vi "DestroyClone.vi"(8 "error in (no error)":errorcluster, 9 "Exit via Stop Module Req?":bool, 10 "Wait for Module to stop?":bool, 11 "ModuleAdmin":refnum<class "ModuleAdmin.lvclass">) -> (0 "error out":errorcluster, 1 "External Launch":bool, 3 "Mod Admin out":refnum<class "ModuleAdmin.lvclass">)   [LabVIEW 2014, in "FGenModule.lvlib"]
uses:
  FGenModule.lvlib
  <userlib>/NIST/ModuleAdminLib/ModuleAdmin/ModuleAdmin.lvclass
  <userlib>/NIST/ModuleAdminLib/ModuleAdmin/ModuleAdmin.lvclass/ModuleAdmin.ctl
  <userlib>/NIST/ModuleAdminLib/ModuleAdmin/Accessors/Read CloneRegRef.vi
  <userlib>/NIST/ModuleAdminLib/CloneRegistration/CloneRegistration.lvclass
  <userlib>/NIST/ModuleAdminLib/ModuleAdminBase/ModuleAdminBase.lvclass
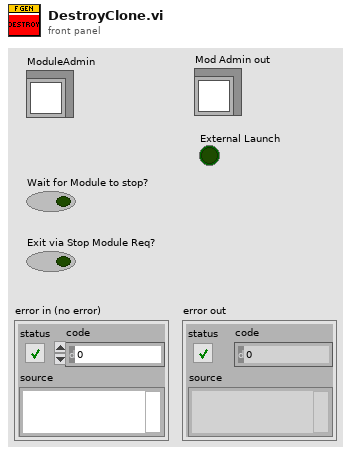
[diagram p1: front panel]
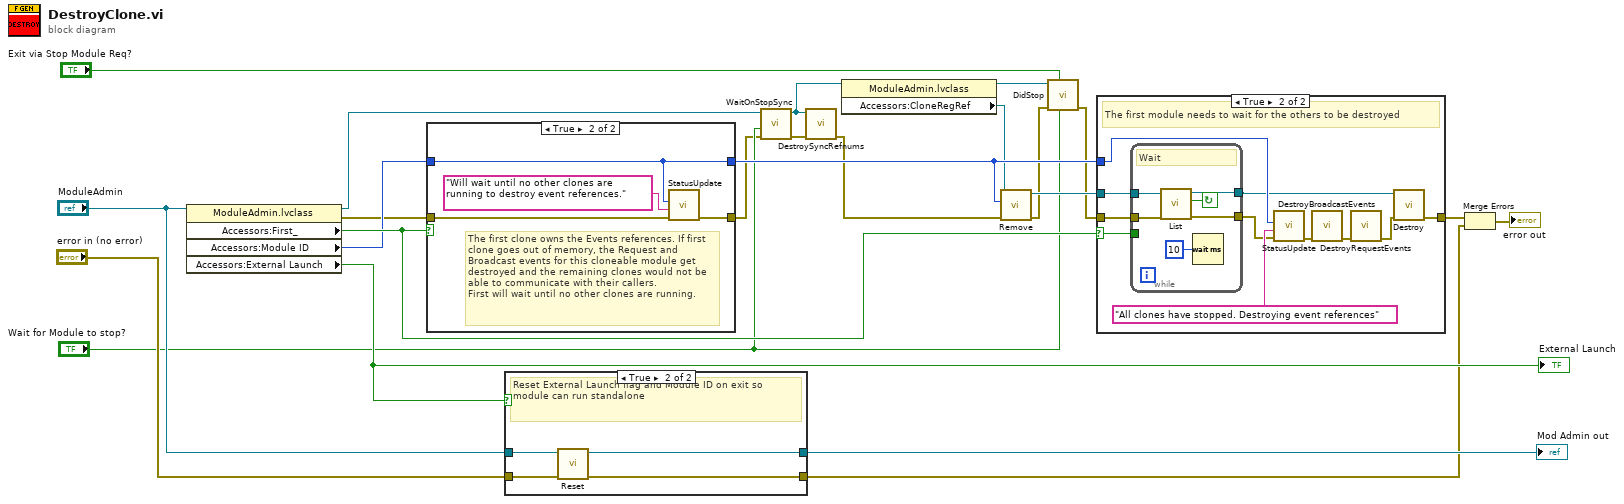
[diagram p0: block diagram]
diagram:
  n1 = property class="ModuleAdmin.lvclass"(reference="ModuleAdmin") -> (reference out=w8:refnum<class "ModuleAdmin.lvclass">, error out=w5:errorcluster, "Accessors:First_"=w23:bool, "Accessors:Module ID"=w15:i32, "Accessors:External Launch"=w20:bool)  [unwired: 1 in]
  "External Launch" <- w20
  n2 = case shown="True" w23 {
    tunnel: w5 -> [w25 w29]
    tunnel: w15 -> [w24 w26]
    tunnel: [w25 w27] -> w6
    tunnel: [w24 w26] -> w22
    frame False {
    }
    frame True {
      # "The first clone owns the Events references. If first clone goes out of memory, the Request and Broadcast events for this cloneable module get destroyed and the remaining clones would not be able to communicate with their callers.\nFirst will wait until no other clones are running."
      n3 = call "StatusUpdate.vi"("error in (no error)"=w29, "Status"="Will wait until no other clones are running to destroy event references." ("format string"), "ModuleID"=w26) -> ("error out"=w27:errorcluster)  [unwired: 8 in]
    }
  }
  n4 = case shown="True" w20 {
    tunnel: "error in (no error)" -> [w30 w35]
    tunnel: "ModuleAdmin" -> [w31 w34]
    tunnel: [w31 w33] -> w18
    tunnel: [w30 w32] -> w16
    frame False {
    }
    frame True {
      # "Reset External Launch flag and Module ID on exit so module can run standalone"
      n5 = call <userlib>:"Reset.vi"("error in (no error)"=w35, "Mod Admin in"=w34) -> ("error out"=w32:errorcluster, "Mod Admin out"=w33:refnum<class "ModuleAdmin.lvclass">)  [unwired: 8 in]
    }
  }
  "Mod Admin out" <- w18
  n6 = call <userlib>:"WaitOnStopSync.vi"("error in (no error)"=w6, "WaitForModuleToStop?"="Wait for Module to stop?", "ModuleAdmin"=w8) -> ("error out"=w21:errorcluster, "ModuleAdmin"=w7:refnum<class "ModuleAdmin.lvclass">)  [unwired: 7 in]
  n7 = call <userlib>:"DestroySyncRefnums.vi"("error in (no error)"=w21, "ModuleAdmin"=w7) -> ("error out"=w4:errorcluster)  [unwired: 9 in]
  n8 = property class="ModuleAdmin.lvclass"(reference=w7) -> (reference out=w2:refnum<class "ModuleAdmin.lvclass">, "Accessors:CloneRegRef"=w3:refnum<data-value>)  [unwired: 1 in, 1 out]
  n9 = call <userlib>:"Remove.vi"("error in (no error)"=w4, "Module ID"=w22, "CloneRegRef"=w3) -> ("error out"=w11:errorcluster, "CloneRegRef"=w14:refnum<data-value>)  [unwired: 6 in, 1 out]
  n10 = call "DidStop.vi"("Wait for Module to stop?"="Wait for Module to stop?", "Exit via Stop Module Req?"="Exit via Stop Module Req?", "error in (no error)"=w11, "ModuleAdmin"=w2) -> ("error out"=w10:errorcluster)  [unwired: 7 in]
  n11 = case shown="True" w23 {
    selector: w23 -> [_ w46]
    tunnel: w10 -> [w36 w47]
    tunnel: w22 -> [_ w42]
    tunnel: [w36 w38] -> w12
    tunnel: w14 -> [_ w41]
    frame False {
    }
    frame True {
      # "The first module needs to wait for the others to be destroyed"
      n12 = while {
        tunnel: w47 -> [w53]
        tunnel: w46 -> [_]
        tunnel: [w52] -> w40
        tunnel: w41 -> [w49]
        tunnel: [w48] -> w39
        stop <- w51 continue-if-true
        # "Wait"
        n13 = call <userlib>:"List.vi"("error in (no error)"=w53, "CloneRegRef"=w49) -> ("error out"=w52:errorcluster, "Found?"=w51:bool, "CloneRegRef"=w48:refnum<data-value>)  [unwired: 4 in, 3 out]
        n14 = Wait (ms)(milliseconds to wait=u32 10) -> ()  [unwired: 1 out]
      }
      n15 = call "StatusUpdate.vi"("error in (no error)"=w40, "Status"="All clones have stopped. Destroying event references", "ModuleID"=w42) -> ("error out"=w44:errorcluster)  [unwired: 8 in]
      n16 = call "DestroyBroadcastEvents.vi"("error in (no error)"=w44) -> ("error out"=w43:errorcluster)  [unwired: 10 in]
      n17 = call "DestroyRequestEvents.vi"("error in (no error)"=w43) -> ("error out"=w37:errorcluster)  [unwired: 10 in]
      n18 = call <userlib>:"Destroy.vi"("error in (no error)"=w37, "CloneRegRef"=w39) -> ("error out"=w38:errorcluster)  [unwired: 9 in]
    }
  }
  n19 = Merge Errors(w12, w16) -> (→"error out":errorcluster)
